vi "Set Initialization Data - Main UI.vi"(8 "error in":errorcluster, 11 "Head Worker in":refnum<class "Head Worker.lvclass">) -> (0 "error out":errorcluster, 3 "Head Worker out":refnum<class "Head Worker.lvclass">)   [LabVIEW 2019, in "Head Worker.lvclass"]
doc: "In this VI you can set the initialization data of a statically-linked subWorker."
uses:
  Head Worker.lvclass
  Main UI/Initialization Data.ctl
  Main UI/Response Cases.ctl
  <vilib>/addons/_Workers/Library/Case Label.ctl
  Head Worker.lvclass/Head Worker.ctl
  Main UI/Main UI.lvclass
  C:/Program Files (x86)/National Instruments/LabVIEW 2019/vi.lib/addons/_Workers/Library/Classes/Worker/Worker.lvclass
  <vilib>/addons/_Workers/Library/Workers.lvlib
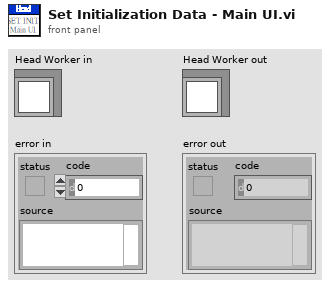
[diagram p1: front panel]
types:
  T1 = typedef "Main UI.lvclass/Initialization Data.ctl" = cluster{"Response Cases":T2}
  T2 = typedef "Main UI.lvclass/Response Cases.ctl" = cluster{"Placeholder - Can be deleted":string, "Start Motor":T3}
  T3 = typedef "Workers.lvlib/Case Label.ctl" = string
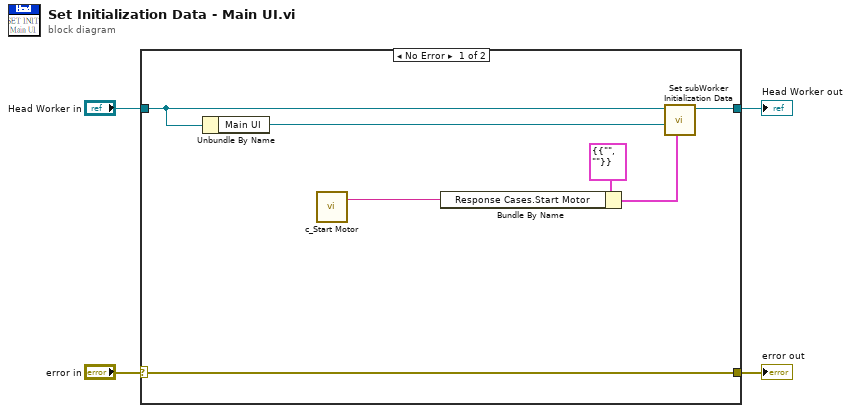
[diagram p0: block diagram]
diagram:
  n1 = case shown="No Error" "error in" {
    selector: "error in" -> [w11 w13]
    tunnel: [w11 w13] -> w3
    tunnel: [w9 w12] -> w2
    tunnel: "Head Worker in" -> [w8 w12]
    frame No Error {
      n2 = Unbundle By Name(w8) -> ("Main UI"=w10:refnum<class "Main UI.lvclass">)
      n3 = call "c_Start Motor.vi"() -> ("Case Label"=w5:T3)  [unwired: 1 in]
      n4 = Bundle By Name(cluster=T1 {"Response Cases"={"Placeholder - Can be deleted"="", "Start Motor"=""}} ("Initialization Data"), "Response Cases.Start Motor"=w5) -> (w6:T1)
      n5 = call-dynamic "Set subWorker Initialization Data.vi"("Initialization Data"=w6, "subWorker"=w10, "Worker"=w8) -> ("Worker out"=w9:refnum<class "Head Worker.lvclass">)  [unwired: 8 in]
    }
    frame Error {
    }
  }
  "error out" <- w3
  "Head Worker out" <- w2
